vi "SetDirection.vi"(8 "error in (no error)":errorcluster caption="entrée d'erreur (pas d'erreur)", 11 "L298N en entrée":refnum<class "L298N.lvclass">) -> (0 "error out":errorcluster caption="sortie d'erreur", 3 "L298N en sortie":refnum<class "L298N.lvclass">)   [LabVIEW 2019, in "L298N.lvclass"]
uses:
  L298N.lvclass
  Action_Type.ctl
  Motor_Type.ctl
panel:
  in  "Moteur":T1
  in  "Action":T2
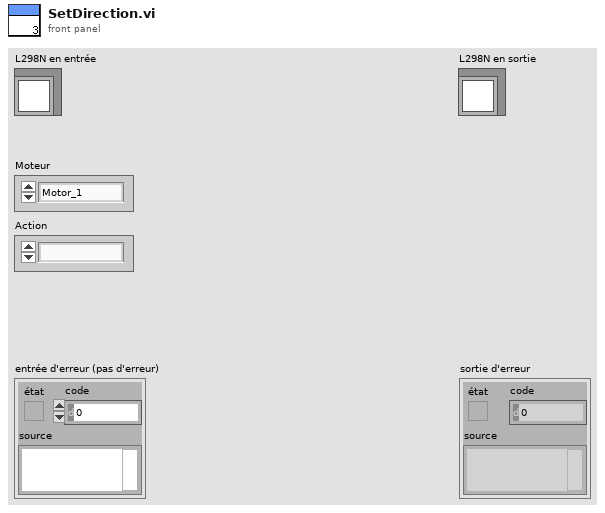
[diagram p1: front panel]
types:
  T1 = typedef "L298N.lvclass/Motor_Type.ctl" = enum16{"Motor_1", "Motor_2", ""}
  T2 = typedef "L298N.lvclass/Action_Type.ctl" = enum16{"", "Up", "Down", "Stop"}
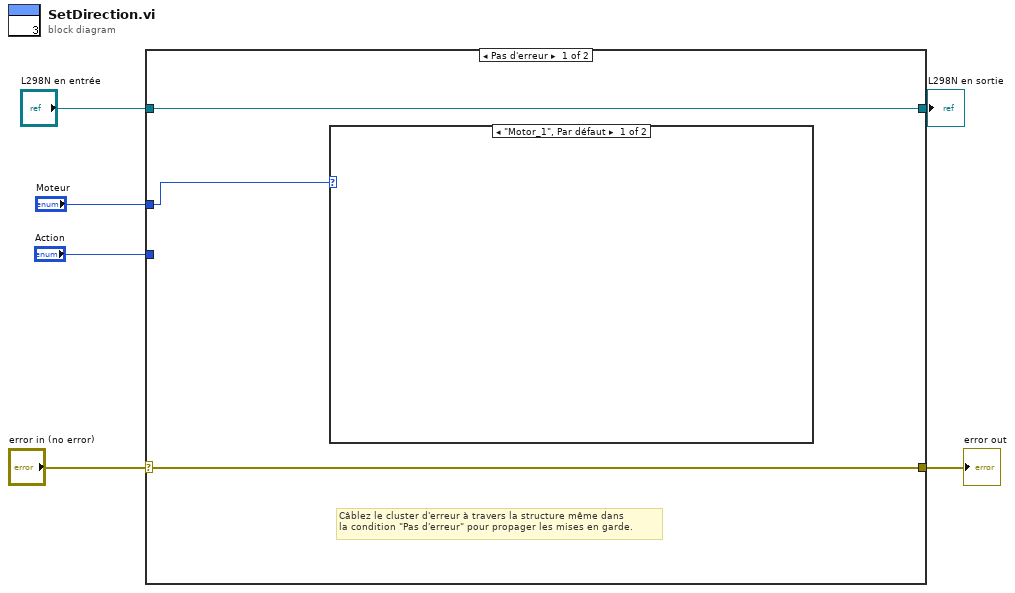
[diagram p0: block diagram]
diagram:
  n1 = case shown="Pas d'erreur" "error in (no error)" {
    selector: "error in (no error)" -> [w8 w11]
    tunnel: [w8 w11] -> w5
    tunnel: [w9 w10] -> w3
    tunnel: "L298N en entrée" -> [w9 w10]
    tunnel: "Moteur" -> [w7 _]
    tunnel: "Action" -> [_ _]
    frame No Error {
      # "Câblez le cluster d'erreur à travers la structure même dans\nla condition \"Pas d'erreur\" pour propager les mises en garde."
      n2 = case shown="\"Motor_1\", Par défaut" w7 {
        frame "Motor_1", Default {
        }
        frame "Motor_2" {
        }
      }
    }
    frame Error {
    }
  }
  "error out" <- w5
  "L298N en sortie" <- w3
